vi "swmm_initialize.vi"(3 "Success msg?":bool, 5 "SWMM Input File (.inp)":path) -> (0 "error out":errorcluster)   [LabVIEW 2014]
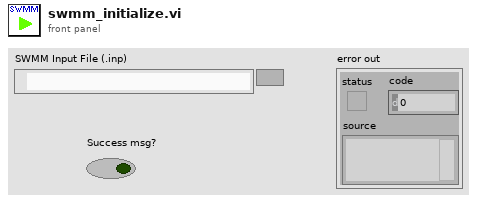
[diagram p1: front panel]
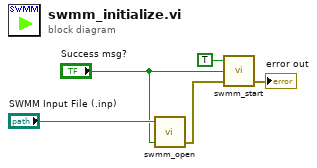
[diagram p0: block diagram]
diagram:
  n1 = call "swmm_open.vi"("Display success msg"="Success msg?", "SWMM Input File (.inp)"="SWMM Input File (.inp)") -> ("error out"=w4:errorcluster)  [unwired: 3 in]
  n2 = call "swmm_start.vi"("error in (no error)"=w4, "Success msg?"="Success msg?", "Write Report?"=TRUE) -> ("error out"=→"error out":errorcluster)  [unwired: 2 in]
